vi "ViconDataAnalysis_pel.vi"(7 "Constants HL":T1={"Frame Points"=[], "Brace Points in P"=[], "QP_lb"=[], "QP_ub"=[], "Q for QP"=[], "nMotors"=0, "QP stopping criteria"={"function tolerance"=1e-08, "parameter tolerance"=1000000.0, "max iterations"=10000, "max function calls"=10000, "gradient tolerance"=1000000.0, "max time (sec)"=-1.0}, "MotorsPos_wrt_Markers"=[], "nMotors 1"=0, "nMotors 2"=0, "MotorsPos_wrt_Markers pel"=[], "Frame Points_pel"=[], "Brace Points in P_pel"=[], "QP_lb pel"=[], "QP_ub pel"=[], "Q for QP pel"=[], "MotorsPos_wrt_Markers knees"=[], "nMotors 3"=0}, 10 "viconData":dbl[](array[numeric])) -> (0 "xyzPlate":dbl[](array[numeric]), 1 "Cn":dbl[](array[numeric]), 2 "CenPt":dbl[](array[numeric]), 3 "StructureMatrix (A)":dbl[][](array[numeric]), 4 "FrameNo (frN)":dbl)   [LabVIEW 2017]
uses:
  typeDef/constants_HL.ctl
  <vilib>/gmath/NumericalOptimization/stopping criteria.ctl
  <vilib>/imath/engines/lvmath2/RunTimeEngine/Managers/WorkSpace/UID Generator.vi
  <vilib>/imath/engines/lvmath2/RunTimeEngine/IndexRead/NIMS V(S).vi
  <instcachedir>/0/NIMS V(S)_0488751826AF41519A22953C041130DC.lvgen/NIMS V(S)_0488751826AF41519A22953C041130DC_000.vi
  <vilib>/imathl/engines/lvmath/Functions/Error Handling/Create Error.vi
  <vilib>/imath/engines/lvmath2/RunTimeEngine/IndexRead/NIMS V(R2).vi
  <instcachedir>/0/NIMS V(R2)_C76619605A0E4E9F8B2FA9389712AC47.lvgen/NIMS V(R2)_C76619605A0E4E9F8B2FA9389712AC47_000.vi
  <vilib>/imath/engines/lvmath2/RunTimeEngine/BuiltInFunctions/transpose/NIMS_transpose(GM).vi
  <instcachedir>/0/NIMS_transpose(GM)_822C4B39CC3F4B34B360A85316D387F1.lvgen/NIMS_transpose(GM)_822C4B39CC3F4B34B360A85316D387F1_004.vi
  <vilib>/imath/engines/lvmath2/RunTimeEngine/ErrorHandling/NIMS_Create Error From Enums.vi
  <vilib>/imath/engines/lvmath2/RunTimeEngine/RangeToken/NIMS_Range_R2 - Integer.vi
  <instcachedir>/0/NIMS_Range_R2 - Integer_B2C3C6B11D0E4F789E1772ACB483EB02.lvgen/NIMS_Range_R2 - Integer_B2C3C6B11D0E4F789E1772ACB483EB02_000.vi
  <vilib>/imath/engines/lvmath2/RunTimeEngine/CommandStatement/MC_CommandStatement_break.vi
  <vilib>/imath/engines/lvmath2/RunTimeEngine/VariableToken/NIMS_VariableToken_CondDefinedDefinedByReplace.vi
  <instcachedir>/0/NIMS_VariableToken_CondDefinedDefinedByReplace_D162CFFC24174562A9FEA619A91E1A56.lvgen/NIMS_VariableToken_CondDefinedDefinedByReplace_D162CFFC24174562A9FEA619A91E1A56_002.vi
  <vilib>/imath/engines/lvmath2/RunTimeEngine/IndexRead/NIMS M(S,R2).vi
  <instcachedir>/0/NIMS M(S,R2)_45730E4D0DB74D118F715F4F99DCE4D7.lvgen/NIMS M(S,R2)_45730E4D0DB74D118F715F4F99DCE4D7_000.vi
  <vilib>/imath/engines/lvmath2/RunTimeEngine/BuiltInFunctions/transpose/NIMS_transpose(GV).vi
  <instcachedir>/0/NIMS_transpose(GV)_1D76875BF542458FA31D2D0CC3E998C0.lvgen/NIMS_transpose(GV)_1D76875BF542458FA31D2D0CC3E998C0_000.vi
  <vilib>/imath/engines/lvmath2/RunTimeEngine/ArithmeticOperatorToken/NIMS_ArithmeticOperator_multmx(M,CV).vi
  <instcachedir>/0/NIMS_ArithmeticOperator_multmx(M,CV)_C4CEBAC88ACD4FCE9121CEED56911FC5.lvgen/NIMS_ArithmeticOperator_multmx(M,CV)_C4CEBAC88ACD4FCE9121CEED56911FC5_000.vi
  <vilib>/imath/engines/lvmath2/RunTimeEngine/ArithmeticOperatorToken/NIMS_ArithmeticOperator_plus.vi
  <instcachedir>/0/NIMS_ArithmeticOperator_plus_9255C7DA94A9479C92F91DC2DA9A664F.lvgen/NIMS_ArithmeticOperator_plus_9255C7DA94A9479C92F91DC2DA9A664F_003.vi
  <vilib>/imath/engines/lvmath2/RunTimeEngine/IndexReplace/NIMS V(R2)=M.vi
  <instcachedir>/0/NIMS V(R2)=M_1D3C529870EA4DABB13C8A39A016A075.lvgen/NIMS V(R2)=M_1D3C529870EA4DABB13C8A39A016A075_001.vi
  <vilib>/imath/engines/lvmath2/RunTimeEngine/VariableToken/NIMS_VariableToken_CondDefined.vi
  <instcachedir>/0/NIMS_VariableToken_CondDefined_6E7F1EE7F80E48298C84CF05BD736261.lvgen/NIMS_VariableToken_CondDefined_6E7F1EE7F80E48298C84CF05BD736261_004.vi
  <vilib>/imath/engines/lvmath2/RunTimeEngine/RunTimeType/NIMS_RunTimeType_From StrictType (excl LVString).vi
  <instcachedir>/0/NIMS_RunTimeType_From StrictType (excl LVString)_1019F277F0A747EDBCA0F6C52CA54500.lvgen/NIMS_RunTimeType_From StrictType (excl LVString)_1019F277F0A747EDBCA0F6C52CA54500_000.vi
  <vilib>/imath/engines/lvmath2/RunTimeEngine/LocalVariableDefStatement/MC_LocalVariableDefStatement_Display.vi
  <vilib>/imath/engines/lvmath2/RunTimeEngine/BuiltInFunctions/zeros/NIMS_M=zeros(I32,I32).vi
  <instcachedir>/0/NIMS V(S)_0488751826AF41519A22953C041130DC.lvgen/NIMS V(S)_0488751826AF41519A22953C041130DC_002.vi
  <vilib>/imath/engines/lvmath2/RunTimeEngine/BuiltInFunctions/norm/NIMS_norm(GV,DBL).vi
  <instcachedir>/0/NIMS_norm(GV,DBL)_C4C44DD415AC4ADEB89BF1A7EC5973B3.lvgen/NIMS_norm(GV,DBL)_C4C44DD415AC4ADEB89BF1A7EC5973B3_000.vi
  <vilib>/imath/engines/lvmath2/RunTimeEngine/IndexReplace/NIMS M(S,R2)=V.vi
  <instcachedir>/0/NIMS M(S,R2)=V_7A6CBA24A40E4522B17742971865BE90.lvgen/NIMS M(S,R2)=V_7A6CBA24A40E4522B17742971865BE90_000.vi
  <vilib>/imath/engines/lvmath2/RunTimeEngine/IndexRead/NIMS M(R2,S).vi
  <instcachedir>/0/NIMS M(R2,S)_56813DCFDD5A484292D2195AF15D2BF5.lvgen/NIMS M(R2,S)_56813DCFDD5A484292D2195AF15D2BF5_000.vi
  <vilib>/imath/engines/lvmath2/RunTimeEngine/IndexRead/NIMS M(S,S).vi
  <instcachedir>/0/NIMS M(S,S)_AC51E74150A542F7991B9634C66F3096.lvgen/NIMS M(S,S)_AC51E74150A542F7991B9634C66F3096_000.vi
  <vilib>/imath/engines/lvmath2/RunTimeEngine/IndexReplace/NIMS M(S,S)=S.vi
  <instcachedir>/0/NIMS M(S,S)=S_490F2BBDD0204024B81939EC402D9A55.lvgen/NIMS M(S,S)=S_490F2BBDD0204024B81939EC402D9A55_000.vi
  <vilib>/imath/engines/lvmath2/RunTimeEngine/Managers/SymbolTable/Clear UID.vi
  <vilib>/imath/engines/lvmath2/RunTimeEngine/NodeEndStatement/NIMS_NodeEndStatement_Output.vi
  <instcachedir>/0/NIMS_NodeEndStatement_Output_53EC0D466D134D7ABD903AC30B43404B.lvgen/NIMS_NodeEndStatement_Output_53EC0D466D134D7ABD903AC30B43404B_002.vi
  <instcachedir>/0/NIMS_NodeEndStatement_Output_53EC0D466D134D7ABD903AC30B43404B.lvgen/NIMS_NodeEndStatement_Output_53EC0D466D134D7ABD903AC30B43404B_005.vi
  <instcachedir>/0/NIMS_NodeEndStatement_Output_53EC0D466D134D7ABD903AC30B43404B.lvgen/NIMS_NodeEndStatement_Output_53EC0D466D134D7ABD903AC30B43404B_001.vi
  <vilib>/imath/engines/lvmath2/RunTimeEngine/ErrorHandling/NIMS_Finalize Error.vi
  <vilib>/imath/engines/lvmath2/RunTimeEngine/Managers/SymbolTable/NIMS_WorkSpace.lvlib
  <vilib>/gmath/NI_Gmath.lvlib
panel:
  out "OB":dbl[][](array[numeric])
  out "uT":dbl[][](array[numeric])
  out "R_o2p":dbl[][](array[numeric])
  out "OB_MK":dbl[][](array[numeric])
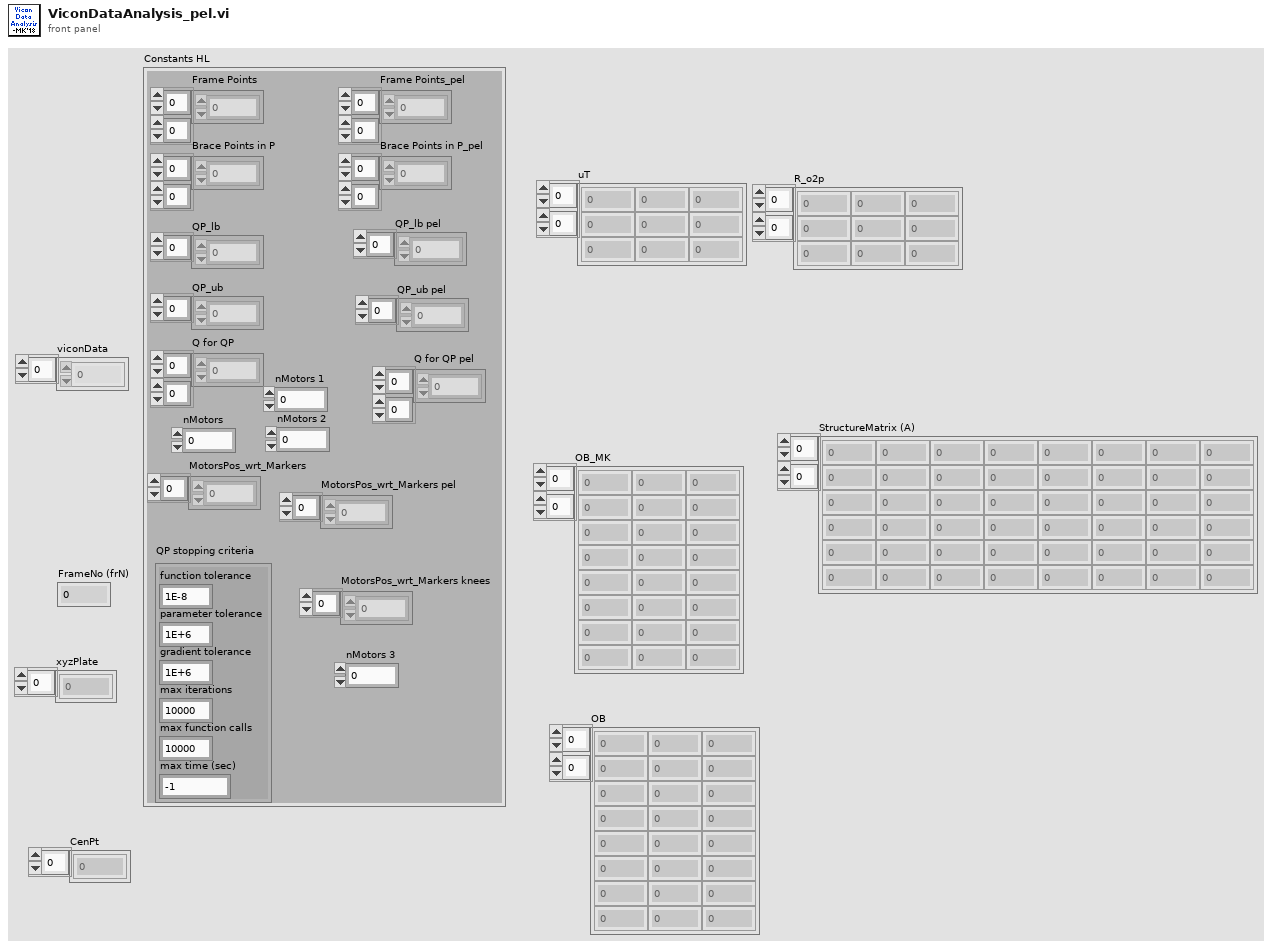
[diagram p1: front panel]
types:
  T1 = typedef "constants_HL.ctl" = cluster{"Frame Points":dbl[][], "Brace Points in P":dbl[][], "QP_lb":dbl[], "QP_ub":dbl[], "Q for QP":dbl[][], "nMotors":i32, "QP stopping criteria":T2, "MotorsPos_wrt_Markers":i32[], "nMotors 1":i32, "nMotors 2":i32, "MotorsPos_wrt_Markers pel":i32[], "Frame Points_pel":dbl[][], "Brace Points in P_pel":dbl[][], "QP_lb pel":dbl[], "QP_ub pel":dbl[], "Q for QP pel":dbl[][], "MotorsPos_wrt_Markers knees":i32[], "nMotors 3":i32}
  T2 = typedef "NI_Gmath.lvlib/stopping criteria.ctl" = cluster{"function tolerance":dbl, "parameter tolerance":dbl, "max iterations":i32, "max function calls":i32, "gradient tolerance":dbl, "max time (sec)":dbl}
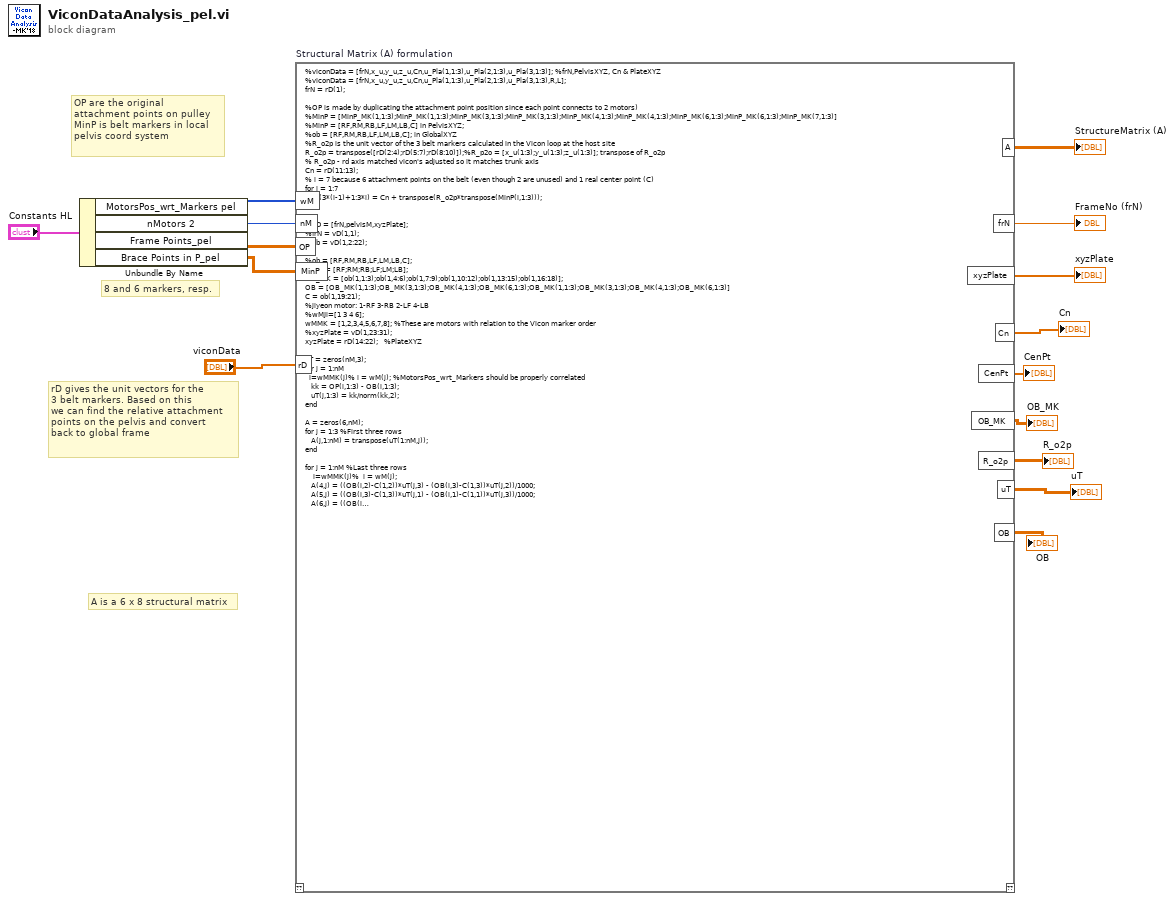
[diagram p0: block diagram]
diagram:
  # "A is a 6 x 8 structural matrix"
  # "8 and 6 markers, resp."
  # "OP are the original\nattachment points on pulley\nMinP is belt markers in local\npelvis coord system"
  # "rD gives the unit vectors for the\n3 belt markers. Based on this\nwe can find the relative attachment\npoints on the pelvis and convert\nback to global frame"
  n1 = Unbundle By Name("Constants HL") -> ("MotorsPos_wrt_Markers pel"=w9:i32[], "nMotors 2"=w11:i32, "Frame Points_pel"=w10:dbl[][], "Brace Points in P_pel"=w8:dbl[][])
  n2 = mathscript code="%viconData = [frN,x_u,y_u,z_u,Cn,u_Pla(1,1:3),u_Pla(2,1:3),u_Pla(3,1:3)]; %frN,PelvisXYZ, Cn & PlateXYZ\n%viconData = [frN,x_u,y_u,z_u,Cn,u_Pla(1,1:3),u_Pla(2,1:3),u_Pla(3,1:3),R,L];\nfrN = rD(1);\n\n%OP is made by duplicating the attachment point position since each point connects to 2 motors)\n%MinP = [MinP_MK(1,1:3);MinP_MK(1,1:3);MinP_MK(3,1:3);MinP_MK(3,1:3);MinP_MK(4,1:3);MinP_MK(4,1:3);MinP_MK(6,1:3);MinP_MK(6,1:3);MinP_MK(7,1:3)]\n%MinP = [RF,RM,RB,LF,LM,LB,C] in PelvisXYZ;\n%ob = [RF,RM,RB,LF,LM,LB,C]; in GlobalXYZ\n%R_o2p is the unit vector of the 3 belt markers calculated in the Vicon loop at the host site\nR_o2p = transpose([rD(2:4);rD(5:7);rD(8:10)]);%R_p2o = [x_u(1:3);y_u(1:3);z_u(1:3)]; transpose of R_o2p\n% R_o2p - rd axis matched vicon's adjusted so it matches trunk axis \nCn = rD(11:13);\n% i = 7 because 6 attachment points on the belt (even though 2 are unused) and 1 real center point (C)\nfor i = 1:7\n   ob(3*(i-1)+1:3*i) = Cn + transpose(R_o2p*transpose(MinP(i,1:3)));\nend\n\n%vD = [frN,pelvisM,xyzPlate];\n%frN = vD(1,1);\n%ob = vD(1,2:22);\n\n%ob = [RF,RM,RB,LF,LM,LB,C];\n%OB = [RF;RM;RB;LF;LM;LB];\nOB_MK = [ob(1,1:3);ob(1,4:6);ob(1,7:9);ob(1,10:12);ob(1,13:15);ob(1,16:18)];\nOB = [OB_MK(1,1:3);OB_MK(3,1:3);OB_MK(4,1:3);OB_MK(6,1:3);OB_MK(1,1:3);OB_MK(3,1:3);OB_MK(4,1:3);OB_MK(6,1:3)]\nC = ob(1,19:21);\n%jiyeon motor: 1-RF 3-RB 2-LF 4-LB\n%wMJi=[1 3 4 6];\nwMMK = [1,2,3,4,5,6,7,8]; %These are motors with relation to the Vicon marker order\n%xyzPlate = vD(1,23:31);\nxyzPlate = rD(14:22);   %PlateXYZ\n\nuT = zeros(nM,3);\nfor j = 1:nM\n  i=wMMK(j)% i = wM(j); %MotorsPos_wrt_Markers should be properly correlated\n   kk = OP(i,1:3) - OB(i,1:3);\n   uT(j,1:3) = kk/norm(kk,2);\nend\n\nA = zeros(6,nM);\nfor j = 1:3 %First three rows\n   A(j,1:nM) = transpose(uT(1:nM,j));\nend\n\nfor j = 1:nM %Last three rows\n    i=wMMK(j)%  i = wM(j);\n   A(4,j) = ((OB(i,2)-C(1,2))*uT(j,3) - (OB(i,3)-C(1,3))*uT(j,2))/1000;\n   A(5,j) = ((OB(i,3)-C(1,3))*uT(j,1) - (OB(i,1)-C(1,1))*uT(j,3))/1000;\n   A(6,j) = ((OB(i,1)-C(1,1))*uT(j,2) - (OB(i,2)-C(1,2))*uT(j,1))/1000;\nend\nCenPt= (rD(23:25)+rD(26:28))/2;" "Structural Matrix (A) formulation"("OP"=w10, "nM"=w11, "wM"=w9, "rD"="viconData", "MinP"=w8) -> ("A"=→"StructureMatrix (A)":dbl[][], "frN"=→"FrameNo (frN)":dbl, "xyzPlate"=→"xyzPlate":dbl[], "Cn"=→"Cn":dbl[], "CenPt"=→"CenPt":dbl[], "OB_MK"=→"OB_MK":dbl[][], "R_o2p"=→"R_o2p":dbl[][], "uT"=→"uT":dbl[][], "OB"=→"OB":dbl[][])  [unwired: 1 in, 1 out]
